vi "read_word.vi"(8 "error in (no error)":errorcluster, 11 "FilePath":string) -> (3 "Text":string)   [LabVIEW 2018]
panel:
  out "error out":errorcluster
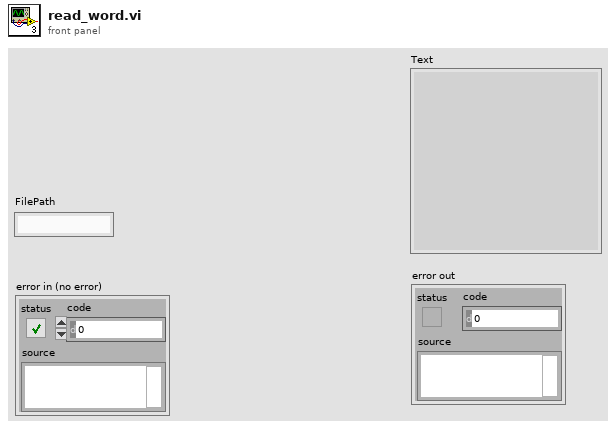
[diagram p1: front panel]
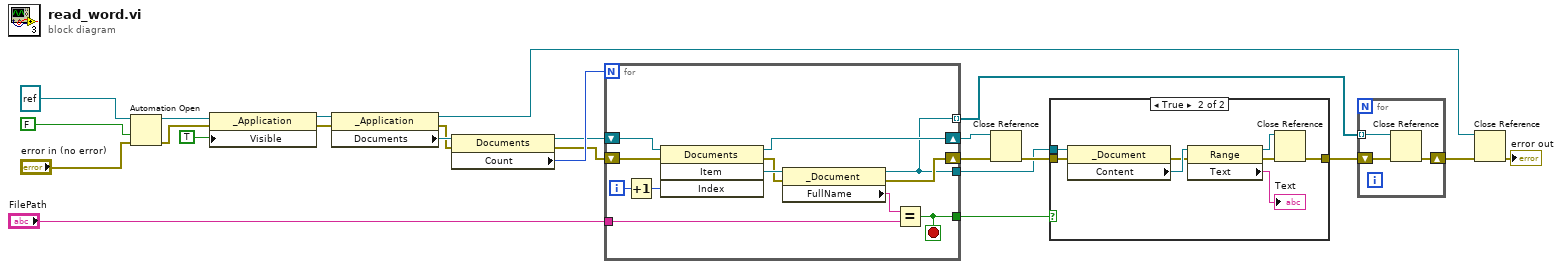
[diagram p0: block diagram]
diagram:
  n1 = Automation Open(error in (no error)="error in (no error)", Automation Refnum=refnum<k7> refnum ("Word._Application"), 9:FALSE ("open new instance (false)")) -> (Automation Refnum=w22:refnum<k7>, error out=w20:errorcluster)  [unwired: 1 in]
  n2 = property class="_Application"(reference=w22, error in=w20, "Visible"=TRUE) -> (reference out=w19:refnum<k7>, error out=w18:errorcluster)
  n3 = property class="_Application"(reference=w19, error in=w18) -> (reference out=w2:refnum<k7>, error out=w6:errorcluster, "Documents"=w8:refnum<k7>)
  n4 = property class="Documents"(reference=w8, error in=w6) -> (reference out=w7:refnum<k7>, error out=w5:errorcluster, "Count"=w12:i32)
  n5 = for {
    N: w12 -> [_]
    tunnel: [w25] -> w13
    shift-right: [w29] -> w16
    shift-left: w5 -> [w35]
    shift-right: [w31] -> w11
    shift-left: w7 -> [w36]
    tunnel: "FilePath" -> [w27]
    tunnel: [w26] -> w3
    tunnel: [w25] -> w1 mode=indexing
    i -> [w34]
    stop <- w26 stop-if-true
    n6 = Increment(x=w34) -> (x+1=w33:i32)
    n7 = invoke class="Documents" method="Item"(reference=w36, error in=w35, "Index"=w33) -> (reference out=w31:refnum<k7>, error out=w30:errorcluster, "Item"=w32:refnum<k7>)  [unwired: 1 in, 1 out]
    n8 = property class="_Document"(reference=w32, error in=w30) -> (reference out=w25:refnum<k7>, error out=w29:errorcluster, "FullName"=w28:string)
    n9 = Equal?(x=w28, y=w27) -> (x = y?=w26:bool)
  }
  n10 = Close Reference(reference=w11, error in (no error)=w16) -> (error out=w15:errorcluster)
  n11 = case shown="True" w3 {
    tunnel: w15 -> [w37 w43]
    tunnel: w13 -> [_ w39]
    tunnel: [w37 w38] -> w10
    frame False {
    }
    frame True {
      n12 = property class="_Document"(reference=w39, error in=w43) -> (error out=w41:errorcluster, "Content"=w45:refnum<k7>)  [unwired: 1 out]
      n13 = property class="Range"(reference=w45, error in=w41) -> (reference out=w42:refnum<k7>, error out=w40:errorcluster, "Text"=→"Text":string)
      n14 = Close Reference(reference=w42, error in (no error)=w40) -> (error out=w38:errorcluster)
    }
  }
  n15 = for {
    shift-right: [w47] -> w9
    shift-left: w10 -> [w48]
    tunnel: w1 -> [w46] mode=indexing
    n16 = Close Reference(reference=w46, error in (no error)=w48) -> (error out=w47:errorcluster)
  }
  n17 = Close Reference(reference=w2, error in (no error)=w9) -> (error out=→"error out":errorcluster)
